vi "replace_cmds_option.vi"(8 "error in (no error)":errorcluster, 11 "String In":string) -> (0 "error out":errorcluster, 3 "String Out":string)   [LabVIEW 2018]
uses:
  <vilib>/regexp/Match Regular Expression.xnode
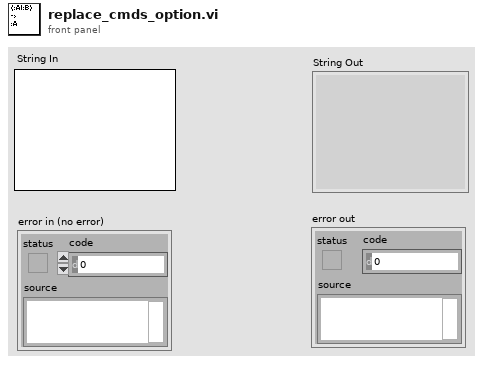
[diagram p1: front panel]
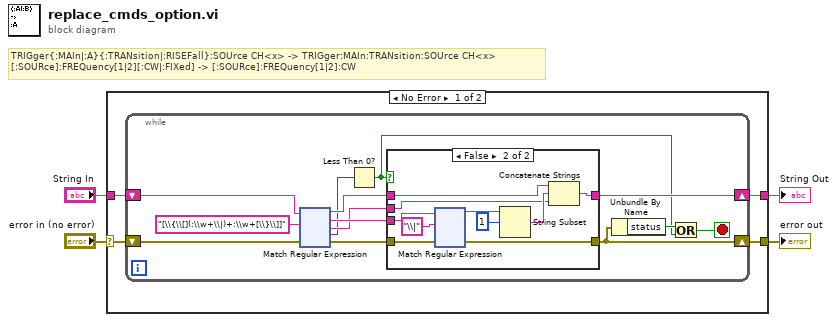
[diagram p0: block diagram]
diagram:
  # "TRIGger{:MAIn|:A}{:TRANsition|:RISEFall}:SOUrce CH<x> -> TRIGger:MAIn:TRANsition:SOUrce CH<x>\n[:SOURce]:FREQuency[1|2][:CW|:FIXed] -> [:SOURce]:FREQuency[1|2]:CW"
  n1 = case shown="No Error" "error in (no error)" {
    selector: "error in (no error)" -> [w6 w256]
    tunnel: "String In" -> [w8 w257]
    tunnel: [w7 w257] -> w3
    tunnel: [w5 w256] -> w1
    frame No Error {
      n2 = while {
        shift-right: [w17] -> w7
        shift-left: w8 -> [w21]
        shift-right: [w12] -> w5
        shift-left: w6 -> [w16]
        stop <- w10 stop-if-true
        n3 = xnode "Match Regular Expression"("input string"=w21, "regular expression"="[\\{\\[](:\\w+\\|)+:\\w+[\\}\\]]", "error in"=w16) -> ("before match"=w18:string, "whole match"=w19:string, "after match"=w14:string, "offset past match"=w13:i32, "error out"=w15:errorcluster)  [unwired: 1 in, 2 out]
        n4 = Less Than 0?(x=w13) -> (x < 0?=w9:bool)
        n5 = case shown="False" w9 {
          tunnel: w19 -> [_ w33]
          tunnel: w18 -> [w23 w31]
          tunnel: [w23 w30] -> w17
          tunnel: w15 -> [w22 w29]
          tunnel: w14 -> [_ w26]
          tunnel: [w22 w24] -> w12
          frame True {
          }
          frame False {
            n6 = xnode "Match Regular Expression"("input string"=w33, "regular expression"="\\|", "error in"=w29) -> ("before match"=w28:string, "error out"=w24:errorcluster)  [unwired: 1 in, 5 out]
            n7 = String Subset(string=w28, offset (0)=1) -> (substring=w27:string)  [unwired: 1 out]
            n8 = Concatenate Strings(w31, w27, w26) -> (w30:string)
          }
        }
        n9 = Unbundle By Name(w12) -> ("status"=w11:bool)
        n10 = Or(x=w11, y=w9) -> (x .or. y?=w10:bool)
      }
    }
    frame Error {
    }
  }
  "String Out" <- w3
  "error out" <- w1
